vi "ResizeProportional.vi"(8 "error in":errorcluster, 10 "Old Bounds":T1, 11 "VI in":refnum<vi>) -> (0 "error out":errorcluster, 2 "Front Panel.PanelBounds":T1)   [LabVIEW 2016]
uses:
  <vilib>/Utility/miscctls.llb/LVRectTypeDef.ctl
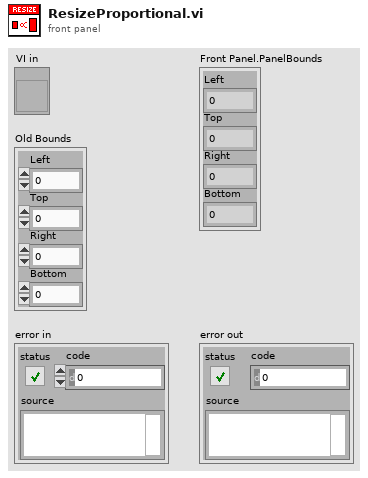
[diagram p1: front panel]
types:
  T1 = typedef "LVRectTypeDef.ctl" = cluster{"Left":i16, "Top":i16, "Right":i16, "Bottom":i16}
  T2 = typedef "LVPointTypeDef.ctl" = cluster{"Horizontal":i16, "Vertical":i16}
  T3 = cluster{"Height":i16, "Width":i16, "Aspect Ratio":dbl}
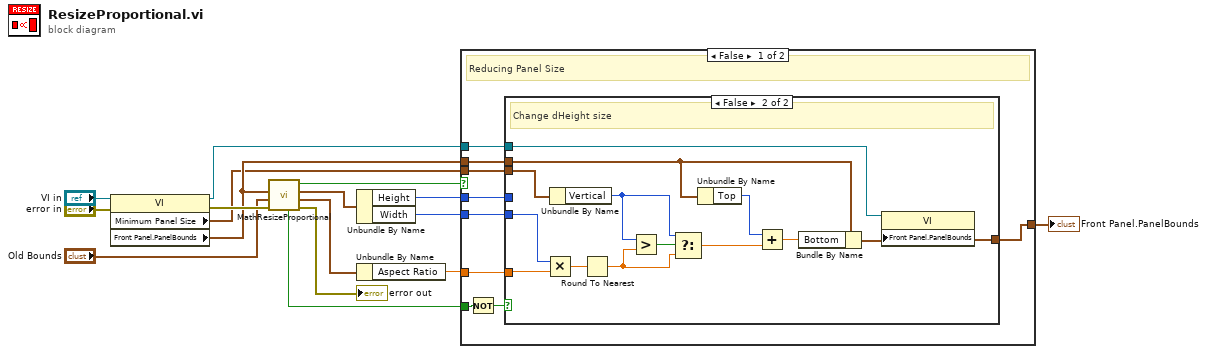
[diagram p0: block diagram]
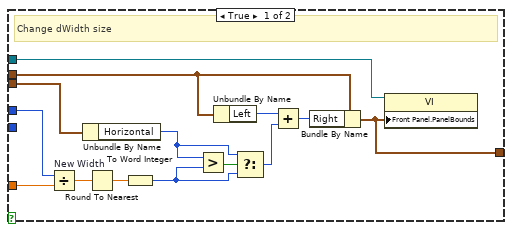
[diagram p2: hidden frame]
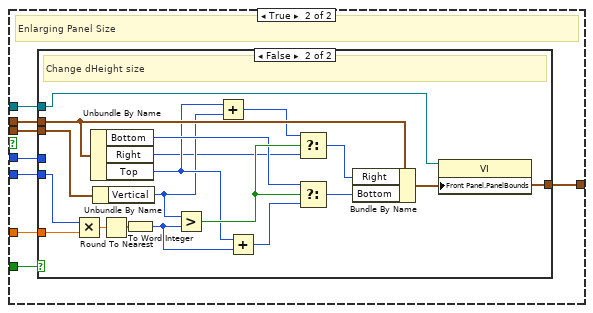
[diagram p3: hidden frame]
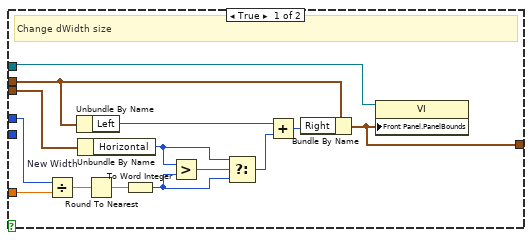
[diagram p4: hidden frame]
diagram:
  n1 = property class="VI"(reference="VI in", error in="error in") -> (reference out=w4:refnum<vi>, error out=w15:errorcluster, "Minimum Panel Size"=w11:T2, "Front Panel.PanelBounds"=w12:T1)
  n2 = call "MathResizeProportional.vi"("error in (no error)"=w15, "Old PanelBounds"="Old Bounds", "New PanelBounds"=w12) -> ("error out"=→"error out":errorcluster, "Old dimensions"=w8:T3, "New dimensions"=w7:T3, "dHeight >= dWidth"=w6:bool, "IncreasingPanel"=w5:bool)  [unwired: 4 in]
  n3 = Unbundle By Name(w7) -> ("Height"=w9:i16, "Width"=w10:i16)
  n4 = Unbundle By Name(w8) -> ("Aspect Ratio"=w14:dbl)
  n5 = case shown="False" w5 {
    tunnel: w4 -> [w25 w60]
    tunnel: [w24 w59] -> w1
    tunnel: w6 -> [w20 w58]
    tunnel: w9 -> [w23 w57]
    tunnel: w10 -> [w22 w56]
    tunnel: w14 -> [w21 w55]
    tunnel: w11 -> [w18 w53]
    tunnel: w12 -> [w17 w54]
    frame False {
      # "Reducing Panel Size"
      n6 = Not(x=w20) -> (.not. x?=w19:bool)
      n7 = case shown="False" w19 {
        tunnel: w25 -> [w31 w45]
        tunnel: w23 -> [w39 _]
        tunnel: w21 -> [w38 w52]
        tunnel: [w34 w49] -> w24
        tunnel: w22 -> [_ w48]
        tunnel: w18 -> [w33 w46]
        tunnel: w17 -> [w32 w47]
        frame True {
          # "Change dWidth size"
          n8 = Divide "New Width"(x=w39, y=w38) -> (x/y=w37:dbl)
          n9 = Unbundle By Name(w33) -> ("Horizontal"=w29:i16)
          n10 = Round To Nearest(number=w37) -> (nearest integer value=w36:dbl)
          n11 = To Word Integer(number=w36) -> (16bit integer=w28:i16)
          n12 = Greater?(x=w29, y=w28) -> (0:w30:bool)
          n13 = Unbundle By Name(w32) -> ("Left"=w35:i16)
          n14 = Select(t=w29, s=w30, f=w28) -> (s? t:f=w27:i16)
          n15 = Add(x=w35, y=w27) -> (x+y=w26:i16)
          n16 = Bundle By Name(cluster=w32, "Right"=w26) -> (w34:T1)
          n17 = property class="VI"(reference=w31, "Front Panel.PanelBounds"=w34) -> ()  [unwired: 1 in, 2 out]
        }
        frame False {
          # "Change dHeight size"
          n18 = Multiply ("New Heigth")(x=w48, y=w52) -> (x*y=w51:dbl)
          n19 = Unbundle By Name(w46) -> ("Vertical"=w43:i16)
          n20 = Round To Nearest(number=w51) -> (nearest integer value=w40:dbl)
          n21 = Greater?(x=w43, y=w40) -> (0:w44:bool)
          n22 = Select(t=w43, s=w44, f=w40) -> (s? t:f=w42:dbl)
          n23 = Unbundle By Name(w47) -> ("Top"=w50:i16)
          n24 = Add(x=w50, y=w42) -> (x+y=w41:dbl)
          n25 = Bundle By Name(cluster=w47, "Bottom"=w41) -> (w49:T1)
          n26 = property class="VI"(reference=w45, "Front Panel.PanelBounds"=w49) -> ()  [unwired: 1 in, 2 out]
        }
      }
    }
    frame True {
      # "Enlarging Panel Size"
      n27 = case shown="False" w58 {
        tunnel: w60 -> [w61 w86]
        tunnel: w57 -> [w74 _]
        tunnel: w55 -> [w73 w91]
        tunnel: [w69 w88] -> w59
        tunnel: w56 -> [_ w87]
        tunnel: w54 -> [w63 w84]
        tunnel: w53 -> [w62 w85]
        frame True {
          # "Change dWidth size"
          n28 = Divide "New Width"(x=w74, y=w73) -> (x/y=w72:dbl)
          n29 = Unbundle By Name(w63) -> ("Left"=w70:i16)
          n30 = Unbundle By Name(w62) -> ("Horizontal"=w65:i16)
          n31 = Round To Nearest(number=w72) -> (nearest integer value=w71:dbl)
          n32 = To Word Integer(number=w71) -> (16bit integer=w66:i16)
          n33 = Greater?(x=w65, y=w66) -> (0:w67:bool)
          n34 = Select(t=w65, s=w67, f=w66) -> (s? t:f=w64:i16)
          n35 = Add(x=w70, y=w64) -> (x+y=w68:i16)
          n36 = Bundle By Name(cluster=w63, "Right"=w68) -> (w69:T1)
          n37 = property class="VI"(reference=w61, "Front Panel.PanelBounds"=w69) -> ()  [unwired: 1 in, 2 out]
        }
        frame False {
          # "Change dHeight size"
          n38 = Multiply(x=w87, y=w91) -> (x*y=w90:dbl)
          n39 = Unbundle By Name(w84) -> ("Bottom"=w81:i16, "Right"=w77:i16, "Top"=w79:i16)
          n40 = Unbundle By Name(w85) -> ("Vertical"=w78:i16)
          n41 = Round To Nearest(number=w90) -> (nearest integer value=w89:dbl)
          n42 = To Word Integer(number=w89) -> (16bit integer=w83:i16)
          n43 = Greater?(x=w78, y=w83) -> (0:w92:bool)
          n44 = Add(x=w79, y=w78) -> (x+y=w80:i16)
          n45 = Add(x=w79, y=w83) -> (x+y=w82:i16)
          n46 = Select(t=w80, s=w92, f=w77) -> (s? t:f=w76:i16)
          n47 = Select(t=w81, s=w92, f=w82) -> (s? t:f=w75:i16)
          n48 = Bundle By Name(cluster=w84, "Right"=w76, "Bottom"=w75) -> (w88:T1)
          n49 = property class="VI"(reference=w86, "Front Panel.PanelBounds"=w88) -> ()  [unwired: 1 in, 2 out]
        }
      }
    }
  }
  "Front Panel.PanelBounds" <- w1
